vi "Target Message Reader.vi"(10 "DIO Ref In":T1, 11 "reader url":refnum<k21>) -> (3 "Stop":bool)   [LabVIEW 2018]
uses:
  Messages.ctl
  <vilib>/myRIO/Instrument Drivers/Onboard IO/DIO/typedefs/DIO Reference.ctl
  <vilib>/myRIO/Common/Instrument Driver Framework/Utilities/typedefs/myRIO Generic Hardware Reference.ctl
  <vilib>/myRIO/Common/Instrument Driver Framework/Utilities/typedefs/Hardware Version Enum.ctl
  <vilib>/myRIO/Common/Instrument Driver Framework/Utilities/typedefs/myRIO v1.0 Reference.ctl
  <vilib>/myRIO/Common/Instrument Driver Framework/Utilities/typedefs/Generic FPGA Reference.ctl
  <vilib>/myRIO/Common/Instrument Driver Framework/myRIO v1.0/DIO/typedefs/DIO Channels List.ctl
  <vilib>/myRIO/Common/Instrument Driver Framework/myRIO v1.0/DIO/typedefs/DIO Channels Enum.ctl
  <vilib>/Utility/error.llb/Error Cluster From Error Code.vi
  <vilib>/myRIO/Common/Instrument Driver Framework/myRIO v1.0/DIO/vis/myRIO v1.0 Write DIO.vi
  <vilib>/myRIO/Instrument Drivers/Onboard IO/DIO/DIO.lvlib
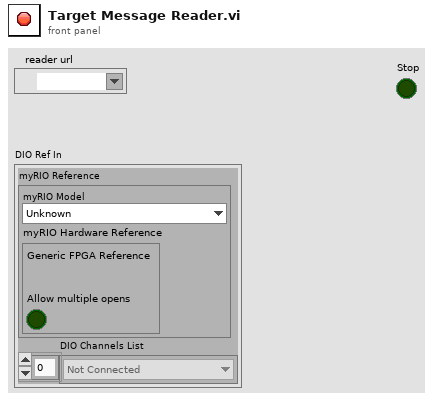
[diagram p1: front panel]
types:
  T1 = typedef "DIO.lvlib/DIO Reference.ctl" = cluster{"myRIO Reference":T2, "DIO Channels List":T6}
  T2 = typedef "myRIO Generic Hardware Reference.ctl" = cluster{"myRIO Model":T3, "myRIO Hardware Reference":T4}
  T3 = typedef "Hardware Version Enum.ctl" = enum16{"Unknown", "myRIO-1900", "myRIO-1950", "roboRIO", "NI ELVIS RIO CM", "ELVIS III"}
  T4 = typedef "myRIO v1.0 Reference.ctl" = cluster{"Generic FPGA Reference":T5, "Allow multiple opens":bool}
  T5 = typedef "Generic FPGA Reference.ctl" = refnum<k20>
  T6 = typedef "DIO Channels List.ctl" = T7[]
  T7 = typedef "DIO Channels Enum.ctl" = enum16{"Not Connected", "C/DIO0", "C/DIO1", "C/DIO2", "C/DIO3", "C/DIO4", "C/DIO5", "C/DIO6", "C/DIO7", "A/DIO0", "A/DIO1", "A/DIO2", "A/DIO3", "A/DIO4", "A/DIO5", "A/DIO6", "A/DIO7", "A/DIO8", "A/DIO9", "A/DIO10", "A/DIO11", "A/DIO12", "A/DIO13", "A/DIO14", "A/DIO15", "A/DIO16", "A/DIO17", "A/DIO18", "A/DIO19", "B/DIO0", "B/DIO1", "B/DIO2", "B/DIO3", "B/DIO4", "B/DIO5", "B/DIO6", "B/DIO7", "B/DIO8", "B/DIO9", "B/DIO10", "B/DIO11", "B/DIO12", "B/DIO13", "B/DIO14", "B/DIO15", "B/DIO16", "B/DIO17", "B/DIO18", "B/DIO19", "LED0", "LED1", "LED2", "LED3", "Button0", "DIO/DIO0", "DIO/DIO1", "DIO/DIO2", "DIO/DIO3", "DIO/DIO4", "DIO/DIO5", "DIO/DIO6", "DIO/DIO7", "DIO/DIO8", "DIO/DIO9", "SPI/CS0", "SPI/CS1", "SPI/CS2", "SPI/CS3", "LED RADIO (Green)", "LED RADIO (Red)", "LED COMM (Green)", "LED COMM (Red)", "LED MODE (Green)", "LED MODE (Red)"}
  T8 = typedef "Messages.ctl" = enum16{"Stop", "Activate/Deactivate Controller", "Log Data", "FF Control Gain Change", "F Thr Change", "dF Thr Change", "Bias Current Change", "Filename Change", "Logging Duration Change", "Phi 1 Change", "Phi End Change", "Phi Remainder Change", "Cutoff Freq Changed", "Control Gain Changed", "Num Phi Param Samples Changed"}
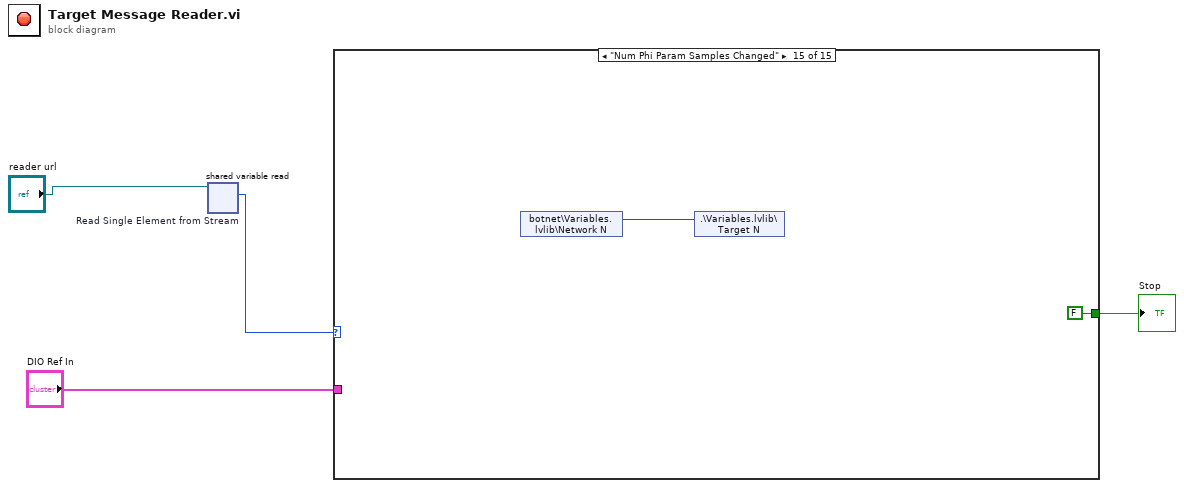
[diagram p0: block diagram]
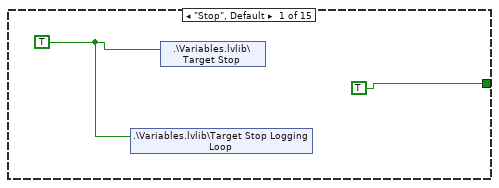
[diagram p2: hidden frame]
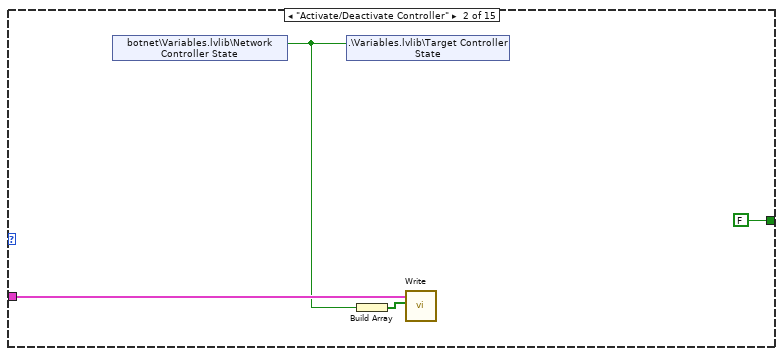
[diagram p3: hidden frame]
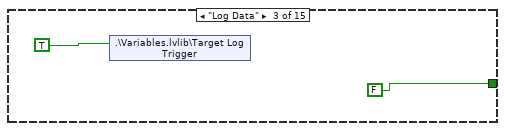
[diagram p4: hidden frame]
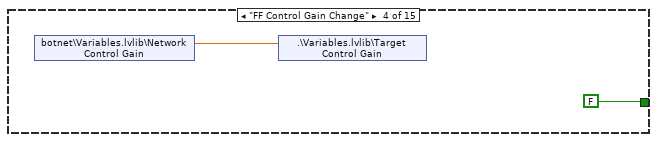
[diagram p5: hidden frame]
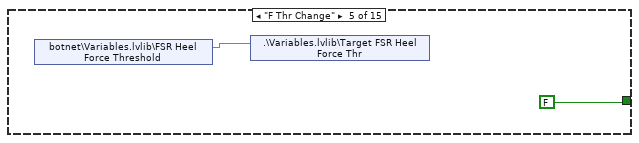
[diagram p6: hidden frame]
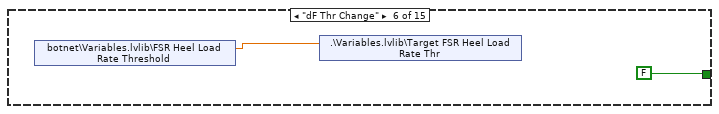
[diagram p7: hidden frame]
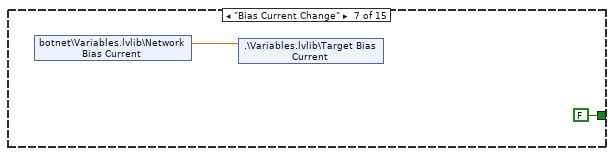
[diagram p8: hidden frame]
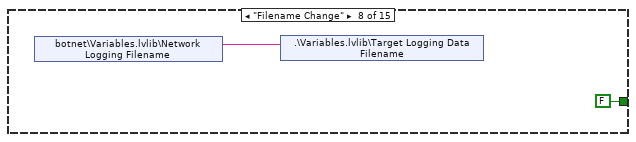
[diagram p9: hidden frame]
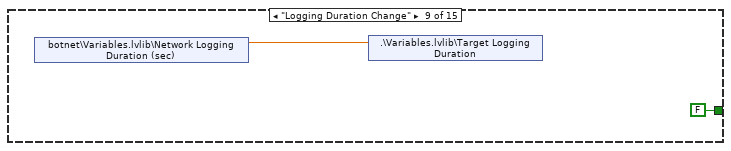
[diagram p10: hidden frame]
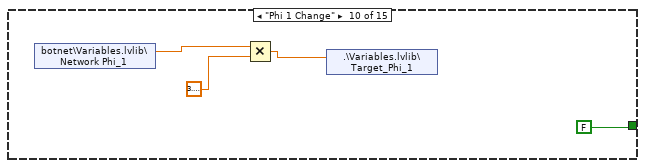
[diagram p11: hidden frame]
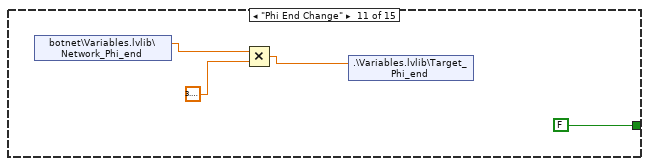
[diagram p12: hidden frame]
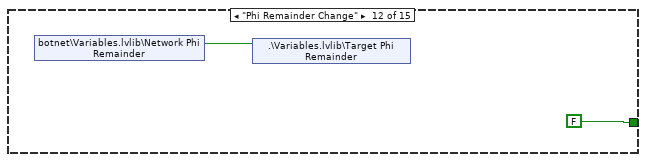
[diagram p13: hidden frame]
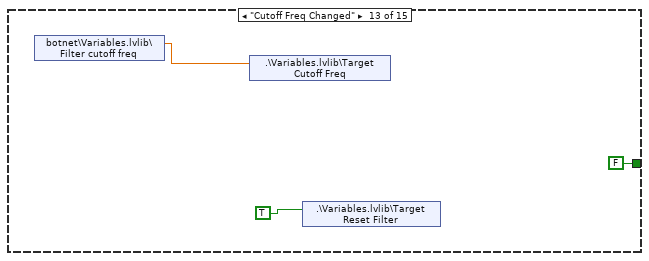
[diagram p14: hidden frame]
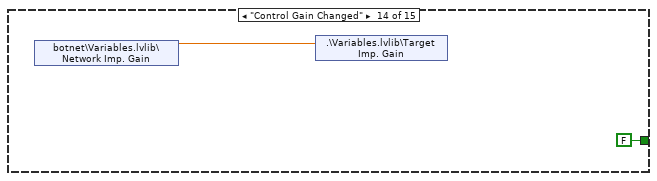
[diagram p15: hidden frame]
diagram:
  n1 = shared-variable-read "Read Single Element from Stream"("reader url") -> (w3:T8)  [unwired: 2 in, 3 out]
  n2 = case shown="\"Num Phi Param Samples Changed\"" w3 {
    tunnel: [TRUE FALSE FALSE FALSE FALSE FALSE FALSE FALSE FALSE FALSE FALSE FALSE FALSE FALSE FALSE] -> w2
    tunnel: "DIO Ref In" -> [_ w9 _ _ _ _ _ _ _ _ _ _ _ _ _]
    frame "Stop", Default {
      w5 = TRUE ("Target Stop")
      n3 = shared-variable ".\\Variables.lvlib\\Target Stop Logging Loop"(w5) -> ()  [unwired: 1 in, 1 out]
      n4 = shared-variable ".\\Variables.lvlib\\Target Stop"(w5) -> ()  [unwired: 1 in, 1 out]
    }
    frame "Activate/Deactivate Controller" {
      n5 = shared-variable "botnet\\Variables.lvlib\\Network Controller State"() -> (w8:bool)  [unwired: 1 in, 1 out]
      n6 = shared-variable ".\\Variables.lvlib\\Target Controller State"(w8) -> ()  [unwired: 1 in, 1 out]
      n7 = Build Array(w8) -> (w7:bool[])
      n8 = call <vilib>:"Write.vi"("Values"=w7, "DIO Ref In"=w9) -> ()  [unwired: 7 in, 2 out]
    }
    frame "Log Data" {
      n9 = shared-variable ".\\Variables.lvlib\\Target Log Trigger"(TRUE ("Target Log Trigger")) -> ()  [unwired: 1 in, 1 out]
    }
    frame "FF Control Gain Change" {
      n10 = shared-variable "botnet\\Variables.lvlib\\Network Control Gain"() -> (w13:dbl)  [unwired: 1 in, 1 out]
      n11 = shared-variable ".\\Variables.lvlib\\Target Control Gain"(w13) -> ()  [unwired: 1 in, 1 out]
    }
    frame "F Thr Change" {
      n12 = shared-variable "botnet\\Variables.lvlib\\FSR Heel Force Threshold"() -> (w16:dbl)  [unwired: 1 in, 1 out]
      n13 = shared-variable ".\\Variables.lvlib\\Target FSR Heel Force Thr"(w16) -> ()  [unwired: 1 in, 1 out]
    }
    frame "dF Thr Change" {
      n14 = shared-variable "botnet\\Variables.lvlib\\FSR Heel Load Rate Threshold"() -> (w18:dbl)  [unwired: 1 in, 1 out]
      n15 = shared-variable ".\\Variables.lvlib\\Target FSR Heel Load Rate Thr"(w18) -> ()  [unwired: 1 in, 1 out]
    }
    frame "Bias Current Change" {
      n16 = shared-variable "botnet\\Variables.lvlib\\Network Bias Current"() -> (w20:dbl)  [unwired: 1 in, 1 out]
      n17 = shared-variable ".\\Variables.lvlib\\Target Bias Current"(w20) -> ()  [unwired: 1 in, 1 out]
    }
    frame "Filename Change" {
      n18 = shared-variable "botnet\\Variables.lvlib\\Network Logging Filename"() -> (w22:string)  [unwired: 1 in, 1 out]
      n19 = shared-variable ".\\Variables.lvlib\\Target Logging Data Filename"(w22) -> ()  [unwired: 1 in, 1 out]
    }
    frame "Logging Duration Change" {
      n20 = shared-variable "botnet\\Variables.lvlib\\Network Logging Duration (sec)"() -> (w23:dbl)  [unwired: 1 in, 1 out]
      n21 = shared-variable ".\\Variables.lvlib\\Target Logging Duration"(w23) -> ()  [unwired: 1 in, 1 out]
    }
    frame "Phi 1 Change" {
      n22 = shared-variable "botnet\\Variables.lvlib\\Network Phi_1"() -> (w26:dbl)  [unwired: 1 in, 1 out]
      n23 = Multiply(x=w26, y=3.141592653589793) -> (x*y=w25:dbl)
      n24 = shared-variable ".\\Variables.lvlib\\Target_Phi_1"(w25) -> ()  [unwired: 1 in, 1 out]
    }
    frame "Phi End Change" {
      n25 = shared-variable "botnet\\Variables.lvlib\\Network_Phi_end"() -> (w31:dbl)  [unwired: 1 in, 1 out]
      n26 = Multiply(x=w31, y=3.141592653589793) -> (x*y=w29:dbl)
      n27 = shared-variable ".\\Variables.lvlib\\Target_Phi_end"(w29) -> ()  [unwired: 1 in, 1 out]
    }
    frame "Phi Remainder Change" {
      n28 = shared-variable "botnet\\Variables.lvlib\\Network Phi Remainder"() -> (w34:bool)  [unwired: 1 in, 1 out]
      n29 = shared-variable ".\\Variables.lvlib\\Target Phi Remainder"(w34) -> ()  [unwired: 1 in, 1 out]
    }
    frame "Cutoff Freq Changed" {
      n30 = shared-variable "botnet\\Variables.lvlib\\Filter cutoff freq"() -> (w37:dbl)  [unwired: 1 in, 1 out]
      n31 = shared-variable ".\\Variables.lvlib\\Target Cutoff Freq"(w37) -> ()  [unwired: 1 in, 1 out]
      n32 = shared-variable ".\\Variables.lvlib\\Target Reset Filter"(TRUE) -> ()  [unwired: 1 in, 1 out]
    }
    frame "Control Gain Changed" {
      n33 = shared-variable "botnet\\Variables.lvlib\\Network Imp. Gain"() -> (w39:dbl)  [unwired: 1 in, 1 out]
      n34 = shared-variable ".\\Variables.lvlib\\Target Imp. Gain"(w39) -> ()  [unwired: 1 in, 1 out]
    }
    frame "Num Phi Param Samples Changed" {
      n35 = shared-variable "botnet\\Variables.lvlib\\Network N"() -> (w41:u32)  [unwired: 1 in, 1 out]
      n36 = shared-variable ".\\Variables.lvlib\\Target N"(w41) -> ()  [unwired: 1 in, 1 out]
    }
  }
  "Stop" <- w2
